vi "receiveCameras.vi"(0 "Vision in":refnum<class "Vision.lvclass">, 1 "Slide":dbl(slide) scale=0.0..10.0, 5 "SSL UDP RX":T1, 7 "Game":refnum<class "Game.lvclass">, 9 "ReplayControlsArray":bool[](array[boolean]), 11 "error in (no error)":errorcluster, 12 "vision?":bool=TRUE) -> (4 "Vision out":refnum<class "Vision.lvclass">, 6 "data camera out":u8[](array[numeric]), 8 "Slide out":dbl(slide) scale=0.0..10.0, 10 "RX":bool, 14 "delay":dbl, 15 "error out":errorcluster)   [LabVIEW 2020, in "Vision.lvclass"]
uses:
  Vision.lvclass
  Controls/vision_control.ctl
  Game_class/Game.lvclass
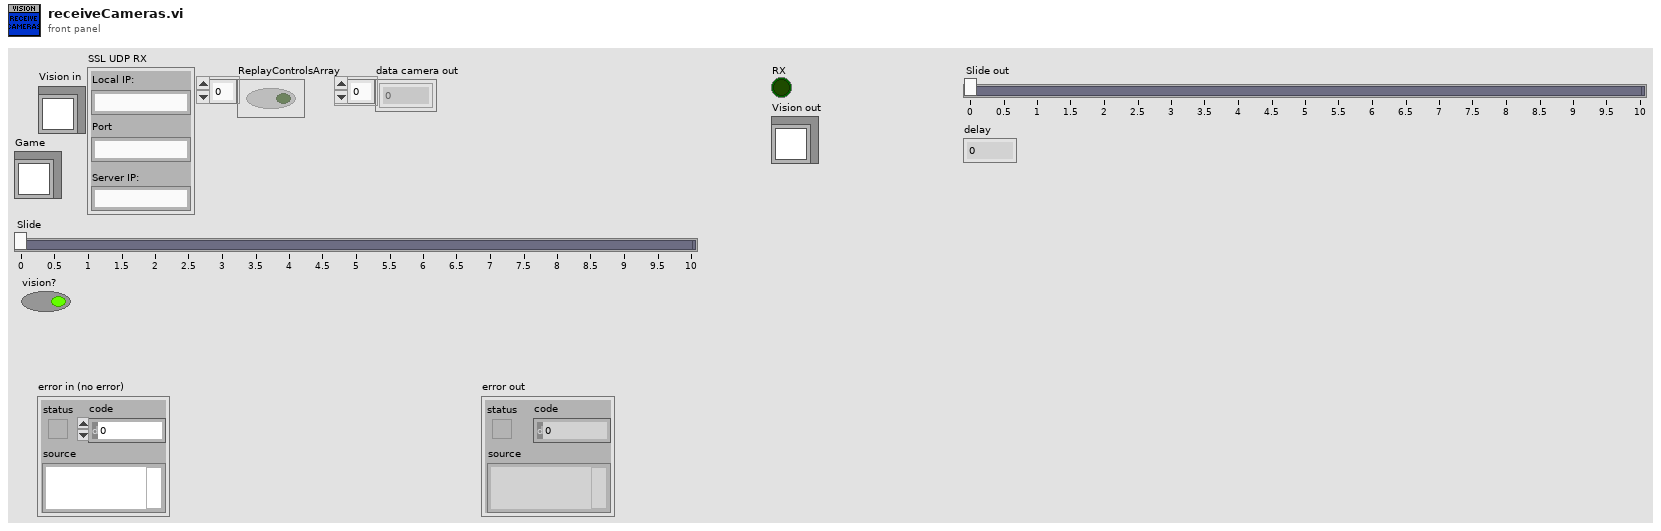
[diagram p1: front panel]
types:
  T1 = typedef "vision_control.ctl" = cluster{"Local IP:":string, "Server IP:":string, "Port":string}
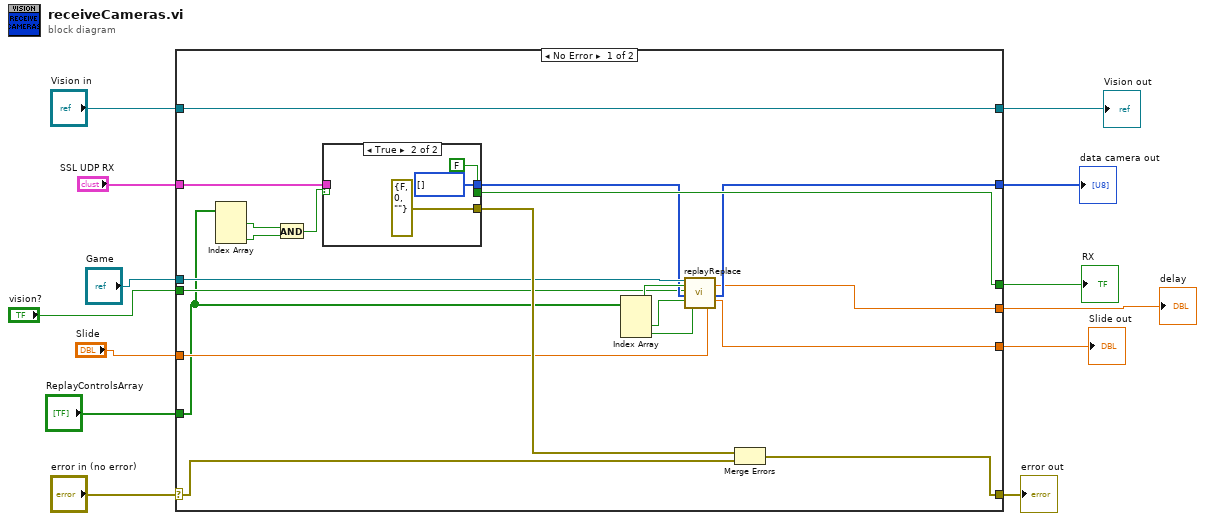
[diagram p0: block diagram]
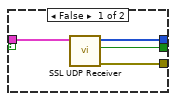
[diagram p2: hidden frame]
diagram:
  n1 = case shown="No Error" "error in (no error)" {
    selector: "error in (no error)" -> [w32 w42]
    tunnel: [w31 w42] -> w12
    tunnel: "Vision in" -> [w29 w41]
    tunnel: [w21 _] -> w10
    tunnel: [w30 _] -> w9
    tunnel: [w29 w41] -> w8
    tunnel: "SSL UDP RX" -> [w28 _]
    tunnel: "Game" -> [w27 _]
    tunnel: "ReplayControlsArray" -> [w17 _]
    tunnel: "Slide" -> [w26 _]
    tunnel: [w20 _] -> w3
    tunnel: [w19 _] -> w2
    tunnel: "vision?" -> [w18 _]
    frame No Error {
      n2 = Index Array(array=w17) -> (element #1=w16:bool, element #3=w15:bool)  [unwired: 3 in, 1 out]
      n3 = And(x=w16, y=w15) -> (x .and. y?=w14:bool)
      n4 = case shown="True" w14 {
        tunnel: [w37 errorcluster {"status"=FALSE, "code"=0, "source"=""} ("error out")] -> w33
        tunnel: [w36 FALSE ("RX")] -> w30
        tunnel: w28 -> [w35 _]
        tunnel: [w34 u8[] [] ("data camera out")] -> w22
        frame False {
          n5 = call "SSL UDP Receiver.vi"("Cluster"=w35) -> ("error out"=w37:errorcluster, "RX"=w36:bool, "data camera out"=w34:u8[])  [unwired: 8 in]
        }
        frame True {
        }
      }
      n6 = Index Array(array=w17) -> (element #1=w25:bool, element #2=w24:bool, element #3=w23:bool)  [unwired: 3 in]
      n7 = call "replayReplace.vi"("Game in"=w27, "On"=w25, "vision?"=w18, "unsigned byte array"=w22, "Play"=w24, "Enable"=w23, "Slide"=w26) -> ("delay"=w19:dbl, "unsigned byte array out"=w21:u8[], "Slide out"=w20:dbl)  [unwired: 7 in, 3 out]
      n8 = Merge Errors(w33, w32) -> (w31:errorcluster)
    }
    frame Error {
    }
  }
  "error out" <- w12
  "data camera out" <- w10
  "RX" <- w9
  "Vision out" <- w8
  "Slide out" <- w3
  "delay" <- w2
